vi "Example_1(SoftwareOnly).vi"() -> ()   [LabVIEW 2011]
uses:
  Ctrls/Configuration.ctl
  Ctrls/ClockDataChannels.ctl
  Ctrls/RegReadWrite.ctl
  <instrlib>/niHWS/nihws.llb/niHWS Store Digital Waveform WDT.vi
panel:
  in  "Data":T1 {"Data" format="%.0x"; "Register" max=31 format="%.0x"; "Slave Address" max=15 format="%.0x"}
  in  "Save Wavform to Disk":bool
  in  "Configuratation":T2={"Samples to Allocate"=10000, "Oversample Factor"=1, "Clock Channel"=enum."0", "Data Channel"=enum."1"} {"Oversample Factor" min=1 max=254; "Samples to Allocate" min=1}
  out "Waveform Graph":digitalwaveform(graph)
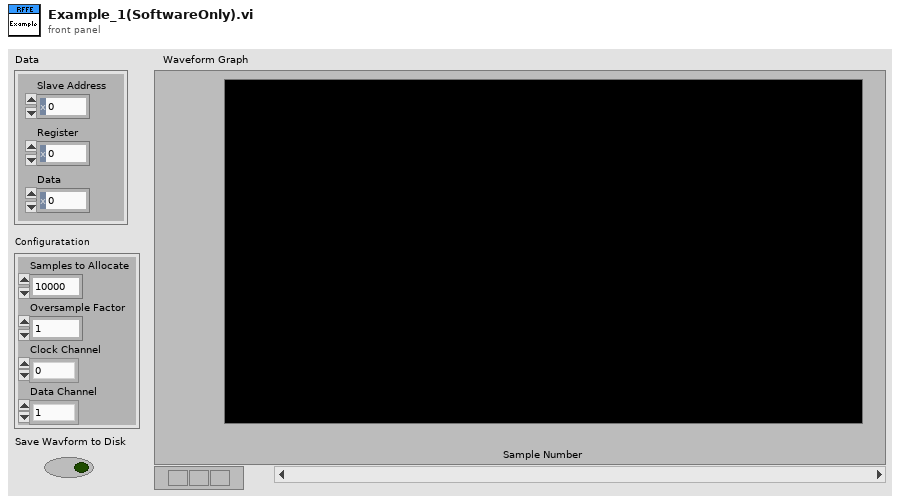
[diagram p1: front panel]
types:
  T1 = typedef "RegReadWrite.ctl" = cluster{"Slave Address":u8, "Register":u8, "Data":u8}
  T2 = typedef "Configuration.ctl" = cluster{"Samples to Allocate":i32, "Oversample Factor":u8, "Clock Channel":T3, "Data Channel":T3}
  T3 = typedef "ClockDataChannels.ctl" = enum16{"0", "1"}
  T4 = typedef "RFFE_Data.ctl" = cluster{"Clock Channel":T3, "Data Channel":T3, "Oversample Factor":u8, "Zero Array":u8[], "One Array":u8[], "Z Array ":u8[], "H Array":u8[], "L Array":u8[], "X Array":u8[], "Toggle (high to low)":u8[]}
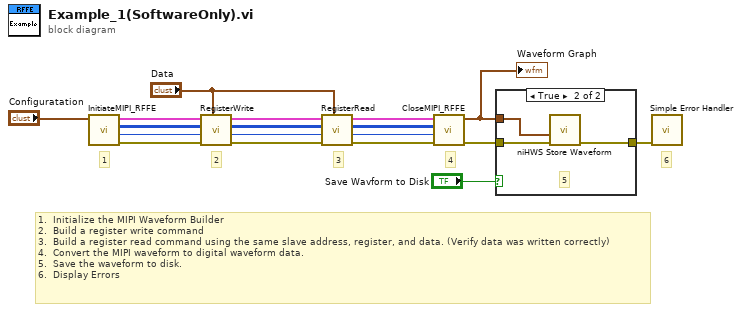
[diagram p0: block diagram]
diagram:
  # "6"
  # "1.  Initialize the MIPI Waveform Builder\n2.  Build a register write command\n3.  Build a register read command using the same slave address, register, and data. (Verify data was written correctly)\n4.  Convert the MIPI waveform to digital waveform data.\n5.  Save the waveform to disk.\n6.  Display Errors"
  # "4"
  # "3"
  # "2"
  # "1"
  n1 = call "InitiateMIPI_RFFE.vi"("Configuratation In"="Configuratation") -> ("error out"=w18:errorcluster, "Number of Samples Out"=w15:i32, "Data Array"=w14:u8[][], "RFFE_Data"=w17:T4)  [unwired: 7 in]
  n2 = call "RegisterWrite.vi"("Write Data"="Data", "error in (no error)"=w18, "Number of Samples In"=w15, "Data Array"=w14, "RFFE_Data"=w17) -> ("error out"=w10:errorcluster, "Number of Samples Out"=w11:i32, "Data Array Out"=w12:u8[][], "Configuratation Out"=w16:T4)  [unwired: 3 in]
  n3 = call "RegisterRead.vi"("Register Read/Write"="Data", "error in (no error)"=w10, "Number of Samples In"=w11, "Data Array"=w12, "RFFE_Data In"=w16) -> ("error out"=w9:errorcluster, "Number of Samples Out out"=w8:i32, "Data Array Out"=w7:u8[][], "RFFE_Data Out"=w6:T4)  [unwired: 2 in, 1 out]
  n4 = call "CloseMIPI_RFFE.vi"("error in (no error)"=w9, "Number of Samples"=w8, "Data Array"=w7, "RFFE_Data"=w6) -> ("error out"=w5:errorcluster, "Digital Waveform"=w4:digitalwaveform)  [unwired: 6 in]
  "Waveform Graph" <- w4
  n5 = case shown="True" "Save Wavform to Disk" {
    tunnel: w5 -> [w19 w22]
    tunnel: w4 -> [_ w21]
    tunnel: [w19 w20] -> w2
    frame False {
    }
    frame True {
      # "5"
      n6 = call-poly <instrlib>:"niHWS Store Waveform.vi"("error in (no error)"=w22, "digital waveform (no data)"=w21) -> ("error out"=w20:errorcluster)  [unwired: 8 in, 1 out]
    }
  }
  n7 = call <vilib>:"Simple Error Handler.vi"("error in (no error)"=w2) -> ()  [unwired: 4 in, 5 out]
